vi "lib next even minute.vi"(10 "time stamp":timestamp) -> (1 "Next Minute":timestamp, 2 "Curr Minute":timestamp)   [LabVIEW 2019]
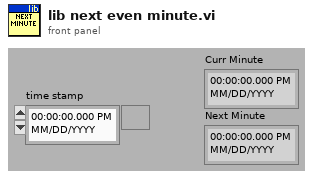
[diagram p1: front panel]
types:
  T1 = typedef "LVDateTimeRec.ctl" = cluster{"fractional second":dbl, "second":i32, "minute":i32, "hour":i32, "day of month":i32, "month":i32, "year":i32, "day of week":i32, "day of year":i32, "DST":i32}
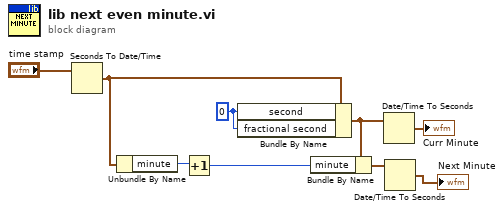
[diagram p0: block diagram]
diagram:
  w7 = 0 ("second")
  n1 = Seconds To Date/Time(time stamp (now)="time stamp") -> (date time rec=w8:T1)  [unwired: 1 in]
  n2 = Unbundle By Name(w8) -> ("minute"=w9:i32)
  n3 = Increment(x=w9) -> (x+1=w4:i32)
  n4 = Bundle By Name(cluster=w8, "second"=w7, "fractional second"=w7) -> (w5:T1)
  n5 = Bundle By Name(cluster=w5, "minute"=w4) -> (w3:T1)
  n6 = Date/Time To Seconds(2:w5) -> (0:→"Curr Minute":timestamp)  [unwired: 1 in]
  n7 = Date/Time To Seconds(2:w3) -> (0:→"Next Minute":timestamp)  [unwired: 1 in]
